vi "Configured Acquisition Trigger 20230130 (Scope1).vi"() -> ()   [LabVIEW 2021]
doc: "Use this VI as a template to design an application that acquires data using advanced triggering logic from the NI PXIe-5170R/5171R."
uses:
  Controls/Queue_Data_Type.ctl
  <instrlib>/HSAI-RIO/Types/v1/Host/Typedefs/Temp Source.ctl
  <vilib>/Analysis/baseanly.llb/Mean (DBL).vi
  <vilib>/FPGAPlugInAG/PXIe-5172 (8CH - 325T)/niLvFpga_Open_PXIe-5172 (8CH - 325T).vi
  <vilib>/rvi/interface/common/dynamic/niFpgaDynamicAddResources.vi
  <vilib>/FPGAPlugInAG/Dynamic/niLvFpga_Close_Dynamic.vi
  <vilib>/rvi/interface/nirviOpenFPGA/nirviOpenFPGA.xnode
  FPGA Bitfiles/Multirecord_Acquisition_20230130.lvbitx
  <vilib>/rvi/interface/nirviCloseFPGA/nirviCloseFPGA.xnode
  Device Session/Device Session.lvclass
  <instrlib>/HSAI-RIO/Types/v1/Host/niHSAI Types v1 Host.lvlib
  <vilib>/Utility/TDMS File Viewer/NI_TDMS File Viewer.lvlib
  <vilib>/Analysis/NI_AALBase.lvlib
panel:
  out "Avgd":dbl format="%0.2f"
  in  "mode":T1(ring)=enum."OR"
  in  "Save":bool
  in  "Levels":T2={"Chan 0 trigger level hi (V)"=0.25, "Chan 0 trigger level lo (V)"=-0.25, " Chan 1 trigger level hi (V)"=0.25, "Chan 1 trigger level lo (V) "=-0.25, " Chan 2 trigger level hi (V)"=0.25, "Chan 2 trigger level lo (V) "=-0.25, " Chan 3 trigger level hi (V)"=0.25, "Chan 3 trigger level lo (V) "=-0.25, " Chan 4 trigger level hi (V)"=0.25, "Chan 4 trigger level lo (V) "=-0.25, " Chan 5 trigger level hi (V)"=0.25, "Chan 5 trigger level lo (V) "=-0.25, " Chan 6 trigger level hi (V)"=0.25, "Chan 6 trigger level lo (V) "=-0.25, " Chan 7 trigger level hi (V)"=0.25, "Chan 7 trigger level lo (V) "=-0.25}
  out "error out 2":errorcluster
  out "appended path":path
  out "Trigger":bool
  out "actual sample rate":dbl=200000000.0 format="%#_6p"
  in  "onboard sample clock rate":dbl(ring)=200000000.0 items=["250 MHz"=250000000.0, "200 MHz"=200000000.0, "150 MHz"=150000000.0]
  in  "impedance":enum8{"Default", "1 mega ohm", "50 ohm"}(ring)
  in  "vertical offset (V)":dbl format="%.2p"
  out "Graph":T3(graph)=[{"relativeX"=-2.5e-06, "sample rate"=5e-09, "data in"=[0.6086595323350694, 0.6082560221354166, 0.606594509548611, 0.6064046223958333, 0.6059061686197916, 0.6071879069010416, 0.6087544759114583, 0.6111043294270833, 0.6109144422743055, 0.6111043294270833, 0.6073777940538194, 0.6095377604166666, 0.6135491265190971, 0.606594509548611, 0.6074727376302083, 0.610012478298611, 0.6123860677083333, 0.6079711914062499, 0.613857693142361, 0.6101311577690971, 0.6120775010850694, 0.6082560221354166, 0.6126708984374999, 0.6097276475694444, 0.6118876139322916, 0.6109144422743055, 0.6097276475694444, 0.6128607855902777, 0.6109144422743055, 0.6095377604166666, 0.6115790473090277, 0.6128607855902777, 0.6139526367187499, 0.6110093858506944, 0.609157986111111, 0.6076863606770833, 0.6129557291666666, 0.6110093858506944, 0.6092529296874999, 0.6120775010850694, 0.6131693522135416, 0.6108194986979166, 0.6126708984374999, 0.6101311577690971, 0.6068793402777777, 0.6114841037326388, 0.6140475802951388, 0.6120775010850694, 0.6108194986979166, 0.6083509657118055, 0.610226101345486, 0.6116977267795138, 0.6115790473090277, 0.6137627495659721, 0.611294216579861, 0.6116977267795138, 0.6105109320746527, 0.6104159884982638, 0.6079711914062499, 0.6094428168402777, 0.6128607855902777, 0.6097276475694444, 0.6101311577690971, 0.6093478732638888, 0.6140475802951388, 0.612575954861111, 0.6087544759114583, 0.6094428168402777, 0.6104159884982638, 0.6115790473090277, 0.6072828504774305, 0.6098225911458333, 0.608944363064236, 0.6110093858506944, 0.6075676812065971, 0.607876247829861, 0.6092529296874999, 0.6094428168402777, 0.610226101345486, 0.6118876139322916, 0.6116977267795138, 0.6086595323350694, 0.6096327039930555, 0.6072828504774305, 0.6073777940538194, 0.6075676812065971, 0.6118876139322916, 0.6074727376302083, 0.6069742838541666, 0.6045294867621527, 0.6111043294270833, 0.6067843967013888, 0.611294216579861, 0.6122911241319444, 0.6107245551215277, 0.6080661349826388, 0.6068793402777777, 0.6088494194878471, 0.6104159884982638, 0.6105109320746527, 0.6124810112847221, 0.6080661349826388, 0.6104159884982638, 0.611294216579861, 0.6111992730034721, 0.6072828504774305, 0.6110093858506944, 0.6111043294270833, 0.6119825575086805, 0.6111043294270833, 0.6110093858506944, 0.6121961805555555, 0.612575954861111, 0.6108194986979166, 0.6104159884982638, 0.6071879069010416, 0.6103210449218749, 0.6103210449218749, 0.6147359212239583, 0.6121961805555555, 0.6114841037326388, 0.6064046223958333, 0.6093478732638888, 0.6081610785590277, 0.610012478298611, 0.6083509657118055, 0.610226101345486, 0.6092529296874999, 0.6120775010850694, 0.6103210449218749, 0.6119825575086805, 0.6126708984374999, 0.6122911241319444, 0.6142374674479166, 0.6115790473090277, 0.6158989800347221, 0.6111043294270833, 0.607876247829861, 0.6103210449218749, 0.608944363064236, 0.6142374674479166, 0.6111043294270833, 0.6123860677083333, 0.609157986111111, 0.6096327039930555, 0.6071879069010416, 0.6084459092881944, 0.6116977267795138, 0.610226101345486, 0.6099175347222221, 0.6082560221354166, 0.6098225911458333, 0.6087544759114583, 0.6098225911458333, 0.6107245551215277, 0.6093478732638888, 0.6111043294270833, 0.6122911241319444, 0.610226101345486, 0.6118876139322916, 0.6081610785590277, 0.6081610785590277, 0.6082560221354166, 0.6040547688802083, 0.6075676812065971, 0.6070929633246527, 0.6083509657118055, 0.6111992730034721, 0.6106058756510416, 0.6114841037326388, 0.6104159884982638, 0.6143324110243055, 0.6117926703559027, 0.6116977267795138, 0.6123860677083333, 0.6122911241319444, 0.6105109320746527, 0.6088494194878471, 0.6123860677083333, 0.6086595323350694, 0.6127658420138888, 0.6090393066406249, 0.6109144422743055, 0.6122911241319444, 0.6094428168402777, 0.6077813042534721, 0.6071879069010416, 0.609157986111111, 0.6092529296874999, 0.6090393066406249, 0.6086595323350694, 0.6050279405381944, 0.6086595323350694, 0.6076863606770833, 0.6061197916666666, 0.606594509548611, 0.6097276475694444, 0.6101311577690971, 0.6088494194878471, 0.610012478298611, 0.6081610785590277, 0.6057162814670138, 0.6113891601562499, 0.6087544759114583, 0.6080661349826388, 0.6113891601562499, 0.6132642957899305, 0.6108194986979166, 0.6114841037326388, 0.609157986111111, 0.6077813042534721, 0.6077813042534721, 0.6146172417534721, 0.6084459092881944, 0.6111992730034721, 0.6080661349826388, 0.6088494194878471, 0.6054077148437499, 0.6085408528645833, 0.6049329969618055, 0.6075676812065971, 0.6104159884982638, 0.6104159884982638, 0.6111992730034721, 0.6096327039930555, 0.6064995659722221, 0.6051228841145833, 0.6067843967013888, 0.602962917751736, 0.6096327039930555, 0.6083509657118055, 0.6070929633246527, 0.6074727376302083, 0.6121961805555555, 0.6122911241319444, 0.6092529296874999, 0.6139526367187499, 0.6120775010850694, 0.6110093858506944, 0.6107245551215277, 0.6132642957899305, 0.607876247829861, 0.607876247829861, 0.6051228841145833, 0.6093478732638888, 0.6070929633246527, 0.6110093858506944, 0.609157986111111, 0.6084459092881944, 0.6097276475694444, 0.6155192057291666, 0.6103210449218749, 0.6086595323350694, 0.6117926703559027, 0.6099175347222221, 0.6132642957899305, 0.6084459092881944, 0.6081610785590277, 0.6067843967013888, 0.6096327039930555, 0.6114841037326388, 0.6119825575086805, 0.6075676812065971, 0.6109144422743055, 0.6129557291666666, 0.610226101345486, 0.6121961805555555, 0.6137627495659721, 0.6111043294270833, 0.609157986111111, 0.6092529296874999, 0.6109144422743055, 0.6064046223958333, 0.6070929633246527, 0.6093478732638888, 0.6097276475694444, 0.6115790473090277, 0.6118876139322916, 0.6106058756510416, 0.6135491265190971, 0.6126708984374999, 0.6079711914062499, 0.6103210449218749, 0.6101311577690971, 0.6105109320746527, 0.6120775010850694, 0.6088494194878471, 0.6097276475694444, 0.6120775010850694, 0.6080661349826388, 0.6108194986979166, 0.6123860677083333, 0.6104159884982638, 0.6120775010850694, 0.6126708984374999, 0.6094428168402777, 0.6120775010850694, 0.6115790473090277, 0.6123860677083333, 0.6104159884982638, 0.6093478732638888, 0.6097276475694444, 0.6098225911458333, 0.6056213378906249, 0.6108194986979166, 0.607876247829861, 0.6111992730034721, 0.6082560221354166, 0.6082560221354166, 0.6106058756510416, 0.608944363064236, 0.6094428168402777, 0.6071879069010416, 0.608944363064236, 0.6062147352430555, 0.6075676812065971, 0.6097276475694444, 0.6114841037326388, 0.6072828504774305, 0.608944363064236, 0.6093478732638888, 0.6084459092881944, 0.6101311577690971, 0.6056213378906249, 0.611294216579861, 0.6083509657118055, 0.6097276475694444, 0.6085408528645833, 0.6116977267795138, 0.6109144422743055, 0.6111043294270833, 0.6098225911458333, 0.613857693142361, 0.6115790473090277, 0.6121961805555555, 0.6096327039930555, 0.6124810112847221, 0.6115790473090277, 0.6116977267795138, 0.610226101345486, 0.6124810112847221, 0.6154242621527777, 0.6110093858506944, 0.6092529296874999, 0.6106058756510416, 0.608944363064236, 0.6104159884982638, 0.6085408528645833, 0.6140475802951388, 0.6097276475694444, 0.609157986111111, 0.6077813042534721, 0.6055026584201388, 0.6095377604166666, 0.6147359212239583, 0.6115790473090277, 0.6111043294270833, 0.6101311577690971, 0.6090393066406249, 0.6103210449218749, 0.611294216579861, 0.6083509657118055, 0.6143324110243055, 0.6121961805555555, 0.6111043294270833, 0.608944363064236, 0.6116977267795138, 0.6120775010850694, 0.610226101345486, 0.6145222981770833, 0.612575954861111, 0.6137627495659721, 0.6104159884982638, 0.6120775010850694, 0.6107245551215277, 0.610226101345486, 0.6134541829427083, 0.6116977267795138, 0.6153293185763888, 0.6103210449218749, 0.6118876139322916, 0.6080661349826388, 0.6124810112847221, 0.6108194986979166, 0.6118876139322916, 0.6106058756510416, 0.6106058756510416, 0.6144273546006944, 0.6127658420138888, 0.612575954861111, 0.608944363064236, 0.6111043294270833, 0.6099175347222221, 0.613644070095486, 0.6150207519531249, 0.6147359212239583, 0.613857693142361, 0.6097276475694444, 0.6118876139322916, 0.6046481662326388, 0.6111043294270833, 0.6098225911458333, 0.608944363064236, 0.607876247829861, 0.611294216579861, 0.6132642957899305, 0.611294216579861, 0.6088494194878471, 0.610226101345486, 0.6087544759114583, 0.6129557291666666, 0.6056213378906249, 0.6119825575086805, 0.6096327039930555, 0.6135491265190971, 0.6062147352430555, 0.608944363064236, 0.6101311577690971, 0.6132642957899305, 0.6090393066406249, 0.6128607855902777, 0.6093478732638888, 0.6105109320746527, 0.6064046223958333, 0.6095377604166666, 0.6085408528645833, 0.610226101345486, 0.6101311577690971, 0.6101311577690971, 0.6126708984374999, 0.6096327039930555, 0.6105109320746527, 0.6121961805555555, 0.6116977267795138, 0.6118876139322916, 0.6096327039930555, 0.6105109320746527, 0.6106058756510416, 0.6096327039930555, 0.6092529296874999, 0.6110093858506944, 0.612575954861111, 0.613644070095486, 0.6094428168402777, 0.6117926703559027, 0.610012478298611, 0.612575954861111, 0.6107245551215277, 0.6111992730034721, 0.6109144422743055, 0.6067843967013888, 0.6051228841145833, 0.6072828504774305, 0.6062147352430555, 0.6080661349826388, 0.6107245551215277, 0.6160888671874999, 0.6103210449218749, 0.6114841037326388, 0.6113891601562499, 0.6104159884982638, 0.609157986111111, 0.6092529296874999, 0.6064995659722221, 0.6106058756510416, 0.6117926703559027, 0.6117926703559027, 0.6141425238715277, 0.6099175347222221, 0.6096327039930555, 0.6127658420138888, 0.6131693522135416, 0.6105109320746527, 0.6119825575086805, 0.6128607855902777, 0.6081610785590277, 0.6085408528645833, 0.6099175347222221, 0.611294216579861, 0.610012478298611, 0.6103210449218749, 0.6071879069010416, 0.611294216579861, 0.6051228841145833, 0.6084459092881944, 0.6082560221354166, 0.6124810112847221, 0.6109144422743055, 0.6108194986979166, 0.6131693522135416, 0.6107245551215277, 0.6119825575086805, 0.6121961805555555, 0.6143324110243055, 0.6114841037326388, 0.6115790473090277, 0.6164923773871527, 0.6106058756510416, 0.6109144422743055, 0.6116977267795138, 0.6084459092881944, 0.6106058756510416, 0.6081610785590277, 0.605312771267361, 0.6081610785590277, 0.6066894531249999, 0.608944363064236, 0.607876247829861, 0.6111043294270833, 0.6109144422743055, 0.6116977267795138, 0.6137627495659721, 0.6117926703559027, 0.6099175347222221, 0.6083509657118055, 0.6094428168402777, 0.6105109320746527, 0.6085408528645833, 0.6107245551215277, 0.610226101345486, 0.6118876139322916, 0.608944363064236, 0.6123860677083333, 0.6099175347222221, 0.610226101345486, 0.6055026584201388, 0.612575954861111, 0.6115790473090277, 0.6109144422743055, 0.6079711914062499, 0.6111043294270833, 0.6072828504774305, 0.610012478298611, 0.6083509657118055, 0.611294216579861, 0.6070929633246527, 0.6119825575086805, 0.6094428168402777, 0.6123860677083333, 0.6115790473090277, 0.6113891601562499, 0.6122911241319444, 0.6099175347222221, 0.6111992730034721, 0.6108194986979166, 0.6110093858506944, 0.6084459092881944, 0.6066894531249999, 0.6057162814670138, 0.6084459092881944, 0.6116977267795138, 0.6090393066406249, 0.610226101345486, 0.6104159884982638, 0.6087544759114583, 0.6094428168402777, 0.6088494194878471, 0.6081610785590277, 0.6119825575086805, 0.6101311577690971, 0.610226101345486, 0.6079711914062499, 0.6119825575086805, 0.6092529296874999, 0.6113891601562499, 0.609157986111111, 0.6064046223958333, 0.6076863606770833, 0.6114841037326388, 0.609157986111111, 0.6116977267795138, 0.6082560221354166, 0.6097276475694444, 0.6093478732638888, 0.6132642957899305, 0.6124810112847221, 0.6123860677083333, 0.6115790473090277, 0.6152343749999999, 0.610226101345486, 0.6103210449218749, 0.6081610785590277, 0.6095377604166666, 0.6054077148437499, 0.6068793402777777, 0.606594509548611, 0.612575954861111, 0.6058112250434027, 0.6124810112847221, 0.6048380533854166, 0.612575954861111, 0.6095377604166666, 0.6135491265190971, 0.6095377604166666, 0.612575954861111, 0.6106058756510416, 0.6117926703559027, 0.6121961805555555, 0.6117926703559027, 0.6086595323350694, 0.6104159884982638, 0.610012478298611, 0.609157986111111, 0.6093478732638888, 0.6111043294270833, 0.6081610785590277, 0.6088494194878471, 0.6088494194878471, 0.6077813042534721, 0.6070929633246527, 0.605312771267361, 0.6068793402777777, 0.6118876139322916, 0.6097276475694444, 0.6116977267795138, 0.6073777940538194, 0.610012478298611, 0.6072828504774305, 0.6090393066406249, 0.6052178276909721, 0.6084459092881944, 0.604244656032986, 0.6098225911458333, 0.6103210449218749, 0.610012478298611, 0.6104159884982638, 0.6134541829427083, 0.6114841037326388, 0.6140475802951388, 0.6126708984374999, 0.607876247829861, 0.6103210449218749, 0.6132642957899305, 0.6106058756510416, 0.6113891601562499, 0.6064995659722221, 0.6111043294270833, 0.6099175347222221, 0.6099175347222221, 0.6094428168402777, 0.6144273546006944, 0.6113891601562499, 0.611294216579861, 0.6124810112847221, 0.6123860677083333, 0.6152343749999999, 0.6124810112847221, 0.6121961805555555, 0.6115790473090277, 0.6141425238715277, 0.6096327039930555, 0.6107245551215277, 0.6081610785590277, 0.6098225911458333, 0.6099175347222221, 0.6057162814670138, 0.6074727376302083, 0.6086595323350694, 0.6123860677083333, 0.6122911241319444, 0.6122911241319444, 0.6103210449218749, 0.6101311577690971, 0.6050279405381944, 0.6057162814670138, 0.608944363064236, 0.6116977267795138, 0.6064995659722221, 0.6126708984374999, 0.606594509548611, 0.608944363064236, 0.606594509548611, 0.6114841037326388, 0.6087544759114583, 0.6093478732638888, 0.6087544759114583, 0.6095377604166666, 0.6064995659722221, 0.6120775010850694, 0.6103210449218749, 0.6147359212239583, 0.6122911241319444, 0.6110093858506944, 0.6088494194878471, 0.6081610785590277, 0.6074727376302083, 0.608944363064236, 0.6055026584201388, 0.6145222981770833, 0.6116977267795138, 0.6123860677083333, 0.610226101345486, 0.6114841037326388, 0.6121961805555555, 0.6135491265190971, 0.6095377604166666, 0.6082560221354166, 0.6067843967013888, 0.610012478298611, 0.6075676812065971, 0.6133592393663194, 0.610012478298611, 0.6145222981770833, 0.6126708984374999, 0.6143324110243055, 0.6122911241319444, 0.6093478732638888, 0.6062147352430555, 0.6059061686197916, 0.6033664279513888, 0.6051228841145833, 0.6071879069010416, 0.6094428168402777, 0.611294216579861, 0.6101311577690971, 0.6095377604166666, 0.6087544759114583, 0.6115790473090277, 0.6147359212239583, 0.6104159884982638, 0.6131693522135416, 0.610012478298611, 0.6081610785590277, 0.6067843967013888, 0.6087544759114583, 0.6061197916666666, 0.6084459092881944, 0.6104159884982638, 0.6119825575086805, 0.6111992730034721, 0.6105109320746527, 0.6086595323350694, 0.6086595323350694, 0.6098225911458333, 0.6111992730034721, 0.6076863606770833, 0.6132642957899305, 0.6084459092881944, 0.6096327039930555, 0.6086595323350694, 0.6124810112847221, 0.607876247829861, 0.6088494194878471, 0.6092529296874999, 0.6123860677083333, 0.6109144422743055, 0.6114841037326388, 0.6126708984374999, 0.6106058756510416, 0.6092529296874999, 0.6084459092881944, 0.6072828504774305, 0.6086595323350694, 0.6062147352430555, 0.6115790473090277, 0.6127658420138888, 0.6150207519531249, 0.6126708984374999, 0.614925808376736, 0.6139526367187499, 0.615993923611111, 0.6079711914062499, 0.6122911241319444, 0.6107245551215277, 0.6153293185763888, 0.6120775010850694, 0.611294216579861, 0.6111992730034721, 0.6130506727430555, 0.6116977267795138, 0.6097276475694444, 0.6066894531249999, 0.6093478732638888, 0.6087544759114583, 0.610012478298611, 0.6098225911458333, 0.6131693522135416, 0.6123860677083333, 0.6124810112847221, 0.6087544759114583, 0.6095377604166666, 0.6077813042534721, 0.6076863606770833, 0.6060011121961805, 0.610012478298611, 0.610012478298611, 0.6103210449218749, 0.6142374674479166, 0.6153293185763888, 0.616207546657986, 0.6110093858506944, 0.6132642957899305, 0.6129557291666666, 0.611294216579861, 0.6103210449218749, 0.6098225911458333, 0.6113891601562499, 0.6094428168402777, 0.6098225911458333, 0.6111992730034721, 0.6128607855902777, 0.6128607855902777, 0.611294216579861, 0.6123860677083333, 0.6127658420138888, 0.6094428168402777, 0.6068793402777777, 0.6068793402777777, 0.6107245551215277, 0.6083509657118055, 0.613644070095486, 0.607876247829861, 0.6115790473090277, 0.6097276475694444, 0.6109144422743055, 0.6101311577690971, 0.6115790473090277, 0.6145222981770833, 0.6116977267795138, 0.6062147352430555, 0.6086595323350694, 0.6107245551215277, 0.6098225911458333, 0.6145222981770833, 0.6119825575086805, 0.6148308648003471, 0.6113891601562499, 0.6070929633246527, 0.6067843967013888, 0.6062147352430555, 0.6090393066406249, 0.6079711914062499, 0.6090393066406249, 0.6101311577690971, 0.6130506727430555, 0.6116977267795138, 0.6103210449218749, 0.6079711914062499, 0.6067843967013888, 0.6086595323350694, 0.6090393066406249, 0.6087544759114583, 0.6090393066406249, 0.6104159884982638, 0.6083509657118055, 0.6124810112847221, 0.6110093858506944, 0.6107245551215277, 0.6120775010850694, 0.6090393066406249, 0.6090393066406249, 0.6099175347222221, 0.6103210449218749, 0.6073777940538194, 0.611294216579861, 0.6086595323350694, 0.6103210449218749, 0.6121961805555555, 0.6109144422743055, 0.6087544759114583, 0.610012478298611, 0.6045294867621527, 0.6064995659722221, 0.6036512586805555, 0.6101311577690971, 0.6092529296874999, 0.6107245551215277, 0.6092529296874999, 0.6148308648003471, 0.6101311577690971, 0.6092529296874999, 0.6062147352430555, 0.6069742838541666, 0.6090393066406249, 0.6070929633246527, 0.6111043294270833, 0.6101311577690971, 0.6114841037326388, 0.6147359212239583, 0.6148308648003471, 0.6143324110243055, 0.6135491265190971, 0.6122911241319444, 0.6106058756510416, 0.6115790473090277, 0.6114841037326388, 0.6130506727430555, 0.6094428168402777, 0.608944363064236, 0.6101311577690971, 0.6077813042534721, 0.6093478732638888, 0.6122911241319444, 0.6094428168402777, 0.6145222981770833, 0.6093478732638888, 0.610012478298611, 0.6114841037326388, 0.6109144422743055, 0.6104159884982638, 0.610226101345486, 0.6097276475694444, 0.6093478732638888, 0.6117926703559027, 0.6146172417534721, 0.610012478298611, 0.611294216579861, 0.6110093858506944, 0.6127658420138888, 0.6131693522135416, 0.6104159884982638, 0.6129557291666666, 0.6095377604166666, 0.6069742838541666, 0.6118876139322916, 0.6093478732638888, 0.6099175347222221, 0.6120775010850694, 0.6119825575086805, 0.6139526367187499, 0.6084459092881944, 0.6092529296874999, 0.6116977267795138, 0.6070929633246527, 0.6086595323350694, 0.610012478298611, 0.6087544759114583, 0.6064046223958333, 0.6108194986979166, 0.6069742838541666, 0.6139526367187499, 0.6088494194878471, 0.6108194986979166, 0.6143324110243055, 0.613644070095486, 0.6088494194878471, 0.6123860677083333, 0.6110093858506944, 0.6153293185763888, 0.6076863606770833, 0.6103210449218749, 0.607876247829861, 0.6119825575086805, 0.6077813042534721, 0.6116977267795138, 0.6106058756510416, 0.6137627495659721, 0.6113891601562499, 0.6093478732638888, 0.6062147352430555, 0.6093478732638888, 0.6123860677083333, 0.6104159884982638, 0.6124810112847221, 0.6155192057291666, 0.613857693142361, 0.6114841037326388, 0.6098225911458333, 0.6127658420138888, 0.6086595323350694, 0.6085408528645833, 0.6054077148437499, 0.6104159884982638, 0.6064995659722221, 0.611294216579861, 0.6092529296874999, 0.612575954861111, 0.6134541829427083, 0.6097276475694444, 0.6099175347222221, 0.6108194986979166, 0.6097276475694444, 0.614925808376736, 0.6132642957899305, 0.6154242621527777, 0.6142374674479166, 0.6120775010850694, 0.6118876139322916, 0.6128607855902777, 0.611294216579861, 0.6103210449218749, 0.6072828504774305, 0.6105109320746527, 0.6058112250434027, 0.607876247829861, 0.6148308648003471, 0.6115790473090277, 0.6101311577690971, 0.6106058756510416, 0.6074727376302083, 0.6107245551215277, 0.6127658420138888, 0.6098225911458333, 0.6095377604166666, 0.6088494194878471, 0.6113891601562499, 0.6153293185763888, 0.6110093858506944, 0.6119825575086805, 0.6080661349826388]}, ...(2 in all)]
  out "fpga temperature (°C)":dbl(slide)=84.16040039062506 scale=0.0..96.0 scale format="%#_6p"
  out "power consumption (W)":dbl(slide)=28.75 scale=0.0..38.25 scale format="%#_6p"
  in  "decimation factor":u16=1
  in  "coupling":enum8{"Default", "DC", "AC"}(ring)
  in  "bandwidth":T4(ring)
  in  "pretrigger samples":u64=50
  in  "number of samples":u64=100
  in  "RIO Device":tag="PXI1Slot8"
  in  "channel(s)":string="0,1"
  in  "vertical range (Vpp)":dbl=1.0 format="%.2p"
  out "error out":errorcluster
  in  "stop":bool
  # "RIO Device"
  # "Trigger Settings"
  # "Vertical Settings"
  # "System Monitor"
  # "Acquisition Settings"
  # "DSP"
  # "Clocking"
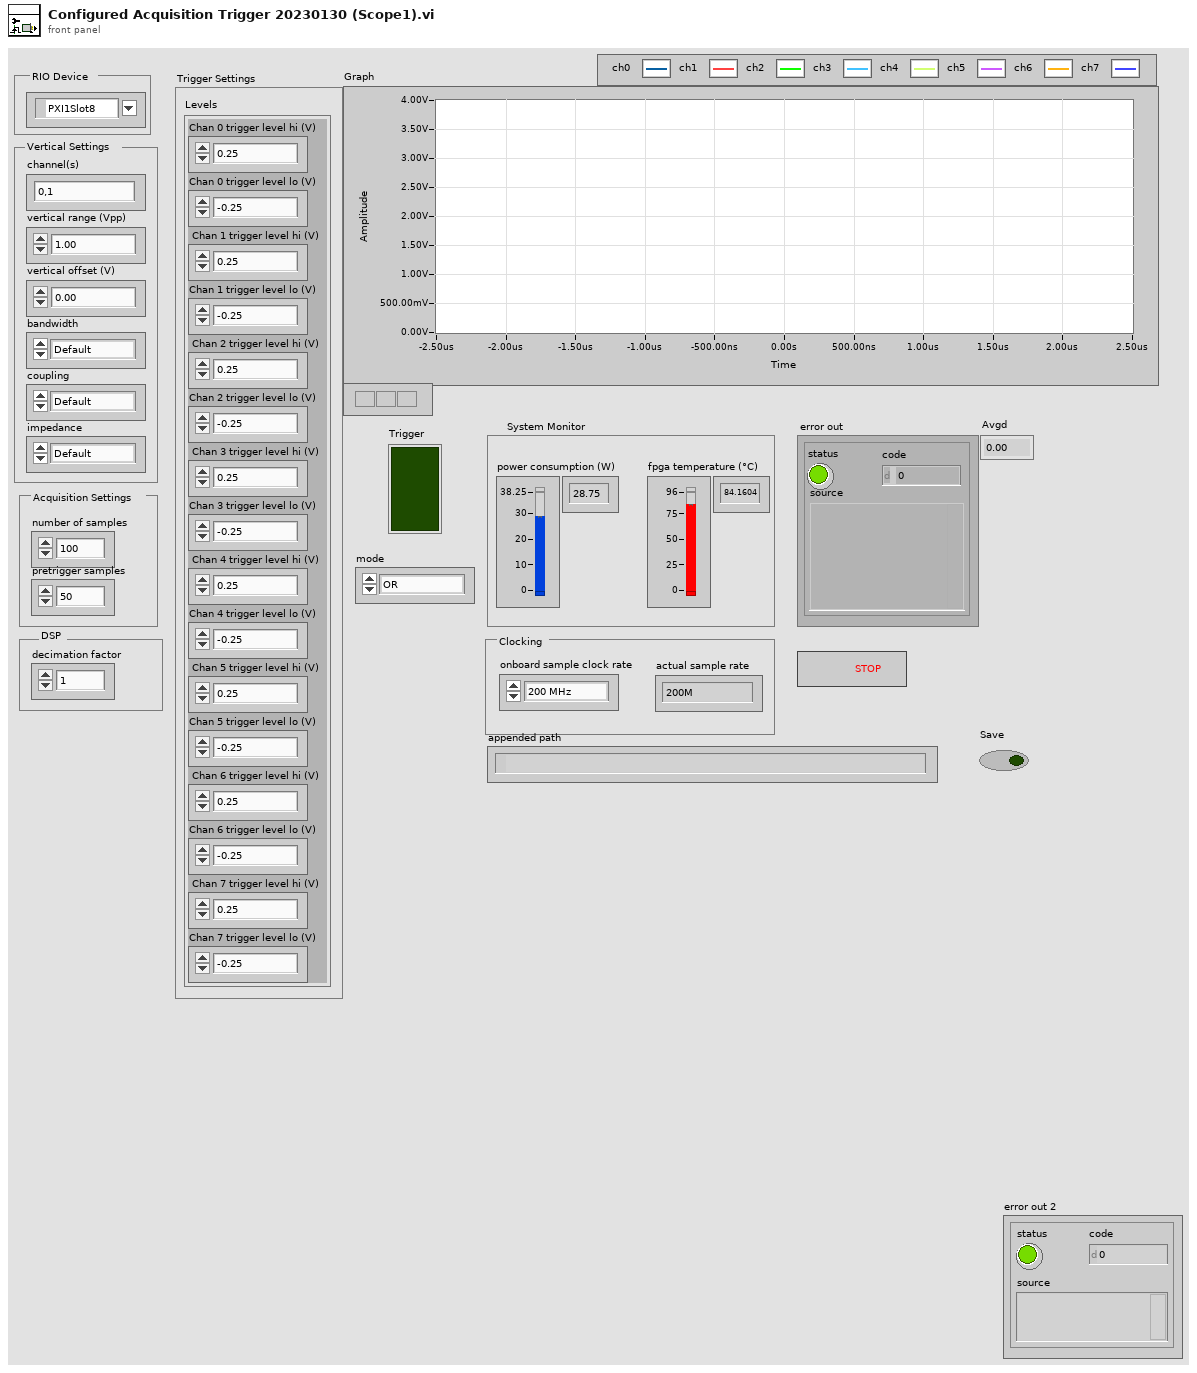
[diagram p1: front panel]
types:
  T1 = enum16{"Immediate", "A", "B", "OR", "AND", "A THEN B", "B THEN A", "High Resolution"}
  T2 = cluster{"Chan 0 trigger level hi (V)":dbl, "Chan 0 trigger level lo (V)":dbl, " Chan 1 trigger level hi (V)":dbl, "Chan 1 trigger level lo (V) ":dbl, " Chan 2 trigger level hi (V)":dbl, "Chan 2 trigger level lo (V) ":dbl, " Chan 3 trigger level hi (V)":dbl, "Chan 3 trigger level lo (V) ":dbl, " Chan 4 trigger level hi (V)":dbl, "Chan 4 trigger level lo (V) ":dbl, " Chan 5 trigger level hi (V)":dbl, "Chan 5 trigger level lo (V) ":dbl, " Chan 6 trigger level hi (V)":dbl, "Chan 6 trigger level lo (V) ":dbl, " Chan 7 trigger level hi (V)":dbl, "Chan 7 trigger level lo (V) ":dbl}
  T3 = cluster{"relativeX":dbl, "sample rate":dbl, "data in":dbl[]}[]
  T4 = enum8{"Default", "Full Bandwidth", "Anti-alias Filter", "80 MHz FIR Filter", "40 MHz FIR Filter", "20 MHz FIR Filter"}
  T5 = typedef "Queue_Data_Type.ctl" = cluster{"date/time string":string, "data":dbl[][]}
  T6 = enum16{"open", "open or create", "create or replace", "create", "open (read-only)"}
  T7 = typedef "niHSAI Types v1 Host.lvlib/Temp Source.ctl" = enum8{"Device Temperature", "Thermal Shutdown Margin", "FPGA Temperature", "FPGA Temperature Limit"}
  T8 = cluster{"date/time string":string, "data":dbl[][]}
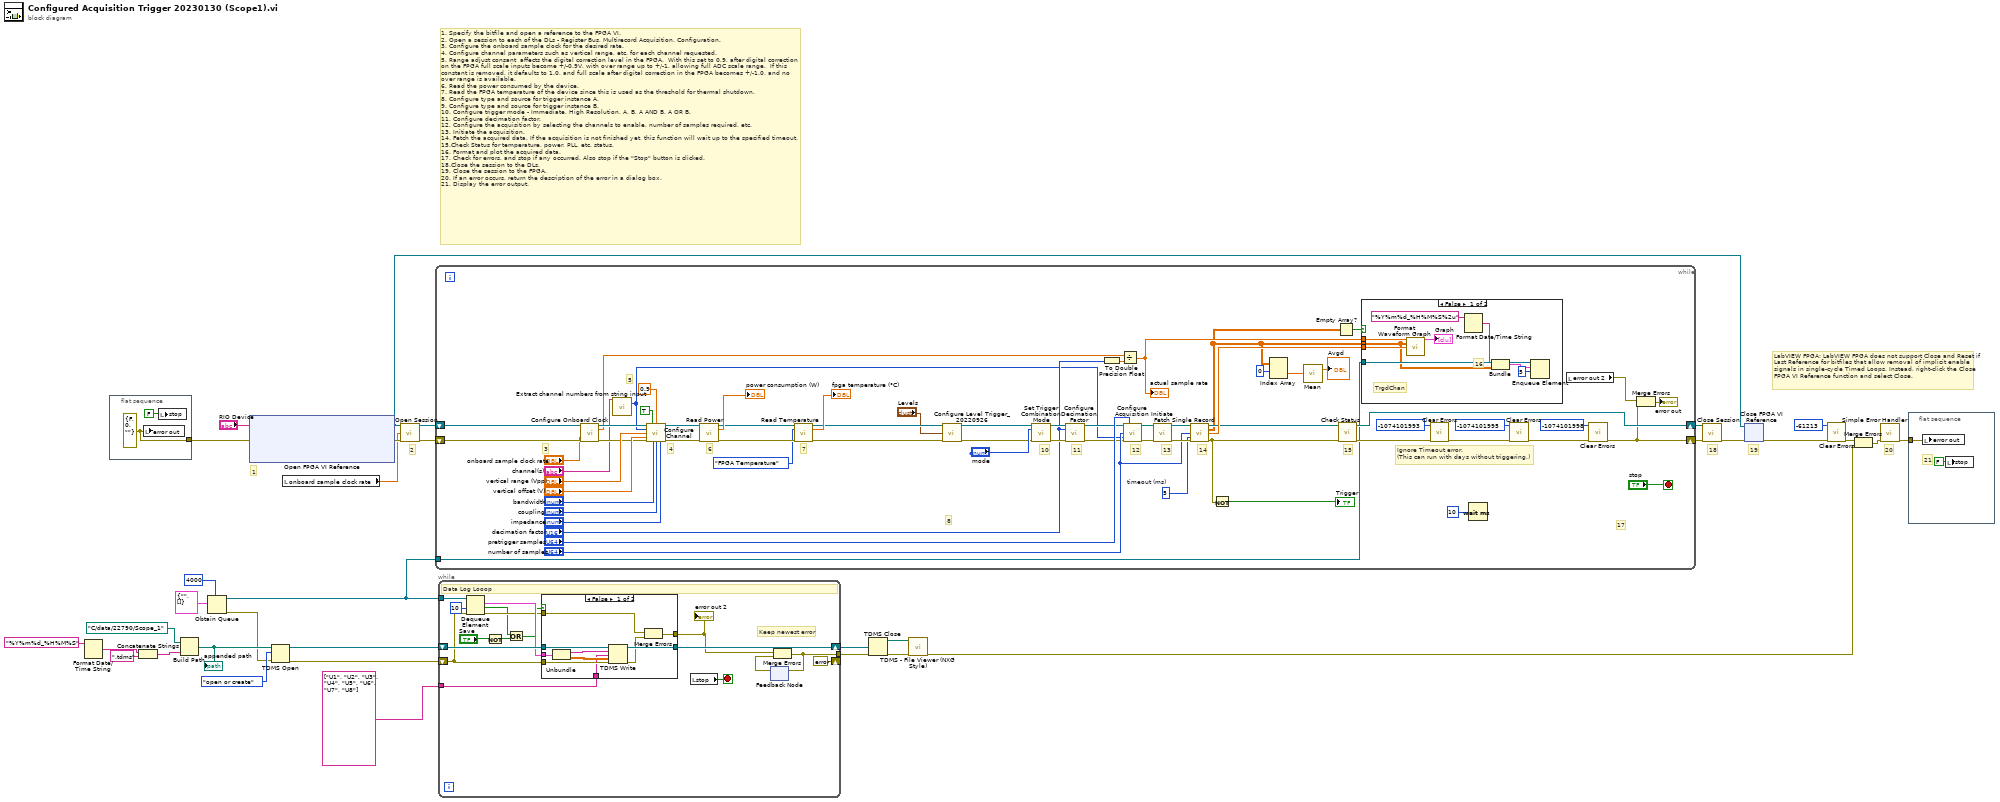
[diagram p0: block diagram]
diagram:
  # "LabVIEW FPGA: LabVIEW FPGA does not support Close and Reset if Last Reference for bitfiles that allow removal of implicit enable signals in single-cycle Timed Loops. Instead, right-click the Close FPGA VI Reference function and select Close."
  # "20"
  # "19"
  # "18"
  # "1. Specify the bitfile and open a reference to the FPGA VI.\n2. Open a session to each of the DLs - Register Bus, Multirecord Acquisition, Configuration.\n3. Configure the onboard sample clock for the desired rate.\n4. Configure channel parameters such as vertical range, etc. for each channel requested.\n5. Range adjust consant  affects the digital correction level in the FPGA.  With this set to 0.9, after digital correction\non the FPGA full scale inputs become +/-0.9V, with over range up to +/-1, allowing full ADC scale range.  If this \nconstant is removed, it defaults to 1.0, and full scale after digital correction in the FPGA becomes +/-1.0, and no\nover range is available.  \n6. Read the power consumed by the device.\n7. Read the FPGA temperature of the device since this is used as the threshold for thermal shutdown.\n8. Configure type and source for trigger instance A.\n9. Configure type and source for trigger instance B.\n10. Configure trigger mode - Immediate, High Resolution, A, B, A AND B, A OR B.\n11. Configure decimation factor.\n12. Configure the acquisition by selecting the channels to enable, number of samples required, etc.\n13. Initiate the acquisition.\n14. Fetch the acquired data. If the acquisition is not finished yet, this function will wait up to the specified timeout.\n15.Check Status for temperature, power, PLL, etc. status. \n16. Format and plot the acquired data.\n17. Check for errors, and stop if any occurred. Also stop if the \"Stop\" button is clicked.\n18.Close the session to the DLs.\n19. Close the session to the FPGA.\n20. If an error occurs, return the description of the error in a dialog box.\n21. Display the error output."
  # "2"
  # "1"
  n1 = Format Date/Time String(time format string (%c)="%Y%m%d_%H%M%S") -> (date/time string=w23:string)  [unwired: 2 in]
  n2 = flat-sequence {
    tunnel: [w36] -> w24
    frame #0 {
      w36 = errorcluster {"status"=FALSE, "code"=0, "source"=""} ("error out")
      n3 = local write "error out"(w36) -> ()
      n4 = local write "stop"(FALSE ("stop")) -> ()
    }
  }
  n5 = Concatenate Strings(w23, ".tdms" ("string")) -> (w22:string)
  n6 = Build Path(base path=path "C:/data/22790/Scope_1", name or relative path=w22) -> (appended path=w19:path)
  "appended path" <- w19
  n7 = Obtain Queue(max queue size (-1, unlimited)=4000, element data type=T5 {"date/time string"="", "data"=[]} ("cluster")) -> (queue out=w12:refnum<queue>, error out=w17:errorcluster)  [unwired: 3 in, 1 out]
  n8 = xnode "Open FPGA VI Reference"("error in"=w24, "resource name"="RIO Device") -> ("FPGA VI Reference Out"=w27:refnum<k20>, "error out"=w29:errorcluster)
  n9 = TDMS Open(8:w17, 10:T6."open or create" ("operation (0:open)"), 11:w19) -> (0:w2:errorcluster, 3:w3:refnum<k34>)  [unwired: 4 in]
  n10 = local read "onboard sample clock rate"() -> (w26:dbl)
  n11 = call "Open Session.vi"("fpga reference in"=w27, "adc clock rate (Hz)"=w26, "error in"=w29) -> ("device session out"=w32:refnum<class "Device Session.lvclass">, "error out"=w31:errorcluster)  [unwired: 11 in]
  n12 = while {
    shift-right: [w49] -> w34
    shift-left: w31 -> [w87]
    shift-right: [w54] -> w33
    shift-left: w32 -> [w88]
    tunnel: w12 -> [w45]
    stop <- "stop" stop-if-true
    w92 = 5  # timeout (ms)
    # "Ignore Timeout error.\n(This can run with days without triggering.)"
    # "4"
    # "5"
    # "7"
    # "6"
    # "15"
    # "11"
    # "3"
    # "17"
    # "10"
    # "8"
    # "14"
    # "13"
    # "12"
    n13 = call "Configure Onboard Clock.vi"("device session in"=w88, "adc clock rate (Hz)"="onboard sample clock rate", "error in"=w87) -> ("device session out"=w86:refnum<class "Device Session.lvclass">, "actual adc clock rate (Hz)"=w78:dbl, "error out"=w85:errorcluster)  [unwired: 9 in, 1 out]
    n14 = call "Extract channel numbers from string input.vi"("channel input"="channel(s)") -> ("array of chans"=w58:u32[])  [unwired: 13 in, 1 out]
    n15 = call "Configure Channel.vi"("device session in"=w86, "enable channel (T)"=TRUE ("enable channel"), "range adjust"=0.9, "channels"=w58, "vertical range (Vpp)"="vertical range (Vpp)", "vertical offset (V)"="vertical offset (V)", "error in"=w85, "bandwidth"="bandwidth", "coupling"="coupling", "impedance"="impedance") -> ("device session out"=w70:refnum<class "Device Session.lvclass">, "error out"=w69:errorcluster)  [unwired: 4 in]
    n16 = call "Read Power.vi"("device session in"=w70, "error in"=w69) -> ("device session out"=w71:refnum<class "Device Session.lvclass">, "power (W)"=→"power consumption (W)":dbl, "error out"=w72:errorcluster)  [unwired: 11 in]
    n17 = call "Read Temperature.vi"("device session in"=w71, "source"=Temp_Source."FPGA Temperature", "error in"=w72) -> ("device session out"=w68:refnum<class "Device Session.lvclass">, "temperature (°C)"=→"fpga temperature (°C)":dbl, "error out"=w67:errorcluster)  [unwired: 10 in]
    n18 = call "Configure Level Trigger_20220926.vi"("device session in"=w68, "Levels"="Levels", "error in"=w67) -> ("device session out"=w57:refnum<class "Device Session.lvclass">, "error out"=w56:errorcluster)  [unwired: 11 in]
    n19 = call "Set Trigger Combination Mode.vi"("device session in"=w57, "mode"="mode", "error in"=w56) -> ("device session out"=w83:refnum<class "Device Session.lvclass">, "error out"=w82:errorcluster)  [unwired: 11 in]
    n20 = call "Configure Decimation Factor.vi"("device session in"=w83, "decimation factor"="decimation factor", "error in"=w82) -> ("device session out"=w80:refnum<class "Device Session.lvclass">, "error out"=w81:errorcluster)  [unwired: 11 in]
    n21 = To Double Precision Float(number="decimation factor") -> (double precision float=w84:dbl)
    n22 = Divide(x=w78, y=w84) -> (x/y=w60:dbl)
    "actual sample rate" <- w60
    n23 = call "Configure Acquisition.vi"("device session in"=w80, "pretrigger samples"="pretrigger samples", "number of samples"="number of samples", "channels to store"=w58, "error in"=w81) -> ("device session out"=w96:refnum<class "Device Session.lvclass">, "error out"=w99:errorcluster)  [unwired: 8 in, 1 out]
    n24 = call "Initiate.vi"("device session in"=w96, "error in"=w99) -> ("device session out"=w97:refnum<class "Device Session.lvclass">, "error out"=w98:errorcluster)  [unwired: 12 in]
    n25 = call "Fetch Single Record.vi"("device session in"=w97, "number of samples"="number of samples", "timeout (ms)"=w92, "error in"=w98) -> ("device session out"=w75:refnum<class "Device Session.lvclass">, "data"=w40:dbl[][], "relativeX (samples)"=w89:dbl, "error out"=w47:errorcluster)  [unwired: 7 in, 1 out]
    n26 = Not(x=w47) -> (.not. x?=→"Trigger":bool)
    n27 = Index Array(array=w40, index (row)=0) -> (element=w38:dbl[])  [unwired: 1 in]
    n28 = call-poly <vilib>:"Mean.vi"("X"=w38) -> ("mean"=→"Avgd":dbl)  [unwired: 1 out]
    n29 = Empty Array?(array=w40) -> (empty?=w46:bool)
    n30 = call "Check Status.vi"("device session in"=w75, "error in"=w47) -> ("device session out"=w54:refnum<class "Device Session.lvclass">, "error out"=w76:errorcluster)  [unwired: 12 in]
    n31 = case shown="False" w46 {
      tunnel: w40 -> [w105 _]
      tunnel: w89 -> [w109 _]
      tunnel: w60 -> [w107 _]
      tunnel: w45 -> [w106 _]
      frame False {
        # "TrgdChan"
        # "16"
        n32 = call "Format Waveform Graph.vi"("sample rate (Hz)"=w107, "data in"=w105, "relativeX (samples)"=w109) -> ("waveform out"=→"Graph":T3)  [unwired: 12 in]
        n33 = Format Date/Time String(time format string (%c)="%Y%m%d_%H%M%S%2u") -> (date/time string=w101:string)  [unwired: 2 in]
        n34 = Bundle("date/time string"=w101, "data"=w105) -> (w102:T8)  [unwired: 1 in]
        n35 = Enqueue Element(queue=w106, element=w102, timeout in ms (-1)=5) -> ()  [unwired: 1 in, 3 out]
      }
      frame True {
        # "No data"
      }
    }
    n36 = call <vilib>:"Clear Errors.vi"("error in (no error)"=w76, "specific error code to clear (0: all)"=-1074101993) -> ("error out"=w52:errorcluster)  [unwired: 4 in, 1 out]
    n37 = Wait (ms)(milliseconds to wait=u32 10) -> ()  [unwired: 1 out]
    n38 = call <vilib>:"Clear Errors.vi"("error in (no error)"=w52, "specific error code to clear (0: all)"=-1074101995) -> ("error out"=w50:errorcluster)  [unwired: 4 in, 1 out]
    n39 = local read "error out 2"() -> (w43:errorcluster)
    n40 = call <vilib>:"Clear Errors.vi"("error in (no error)"=w50, "specific error code to clear (0: all)"=-1074101998) -> ("error out"=w49:errorcluster)  [unwired: 4 in, 1 out]
    n41 = Merge Errors(w43, w49) -> (→"error out":errorcluster)
  }
  n42 = while {
    shift-right: [errorcluster {"status"=FALSE, "code"=0, "source"=""} ("error out")] -> _
    shift-left: w2 -> [w123]
    shift-right: [w125] -> w14
    shift-left: w3 -> [w126]
    tunnel: w12 -> [w124]
    tunnel: [w116] -> w5
    tunnel: string[] ["U1", "U2", "U3", "U4", "U5", "U6", "U7", "U8"] ("Data Log Channel Name") -> [w110]
    stop <- w120 stop-if-true
    # "Keep newest error"
    # "Data Log Looop"
    n43 = Dequeue Element(queue=w124, timeout in ms (-1)=10, error in (no error)=w123) -> (element=w122:T5, timed out?=w114:bool, error out=w121:errorcluster)  [unwired: 1 out]
    n44 = Not(x="Save") -> (.not. x?=w112:bool)
    n45 = Or(x=w114, y=w112) -> (x .or. y?=w113:bool)
    n46 = case shown="False" w113 {
      tunnel: w126 -> [w128 w138]
      tunnel: [w136 w138] -> w125
      tunnel: w123 -> [w135 _]
      tunnel: w122 -> [w134 _]
      tunnel: w121 -> [w133 w137]
      tunnel: [w131 w137] -> w117
      tunnel: w110 -> [w127 _]
      frame False {
        n47 = Unbundle(w134) -> ("date/time string"=w130:string, "data"=w129:dbl[][])
        n48 = TDMS Write(0:w128, 5:w130, 7:w127, 9:w129, 11:w135) -> (4:w136:refnum<k34>, 15:w132:errorcluster)  [unwired: 1 in, 2 out]
        n49 = Merge Errors(w133, w132) -> (w131:errorcluster)
      }
      frame True {
        # "Timed out. No data."
      }
    }
    "error out 2" <- w117
    n50 = local read "stop"() -> (w120:bool)
    n51 = feedback #1() -> (w115:errorcluster)  [unwired: 1 in]
    n52 = Merge Errors(w117, w115) -> (w116:errorcluster)
    n53 = feedback-in #1(w116) -> ()
  }
  n54 = TDMS Close(8:w5, 11:w14) -> (0:w15:errorcluster, 3:w13:path)
  n55 = call <vilib>:"TDMS - File Viewer (NXG Style).vi"("error in"=w15, "file in"=w13) -> ("error out"=w10:errorcluster)  [unwired: 8 in, 1 out]
  n56 = call "Close Session.vi"("device session in"=w33, "error in"=w34) -> ("error out"=w28:errorcluster)  [unwired: 13 in]
  n57 = xnode "Close FPGA VI Reference"("FPGA VI Reference In"=w27, "error in"=w28) -> ("error out"=w7:errorcluster)
  n58 = call <vilib>:"Clear Errors.vi"("error in (no error)"=w7, "specific error code to clear (0: all)"=-61213) -> ("error out"=w6:errorcluster)  [unwired: 4 in, 1 out]
  n59 = Merge Errors(w6, w10) -> (w11:errorcluster)
  n60 = call <vilib>:"Simple Error Handler.vi"("error in (no error)"=w11) -> ("error out"=w25:errorcluster)  [unwired: 4 in, 4 out]
  n61 = flat-sequence {
    tunnel: w25 -> [w140]
    frame #0 {
      # "21"
      n62 = local write "error out"(w140) -> ()
      n63 = local write "stop"(FALSE ("stop")) -> ()
    }
  }
